vi "SphereStripSection.vi"(0 "Ducer":cluster{"radius":dbl, "h":dbl, "l":dbl} {"radius" format="%.2f"; "l" format="%.2f"; "h" format="%.2f"}, 2 "Rotate":dbl format="%.2f") -> (1 "thetas":dbl[](array[numeric]) format="%.2f", 4 "phis":dbl[](array[numeric]) format="%.2f", 6 "x matrix":dbl[][](array[numeric]) format="%.2f", 7 "y matrix":dbl[][](array[numeric]) format="%.2f", 8 "z matrix":dbl[][](array[numeric]) format="%.2f")   [LabVIEW 2022 SP3]
uses:
  <vilib>/Analysis/NI_AALPro.lvlib
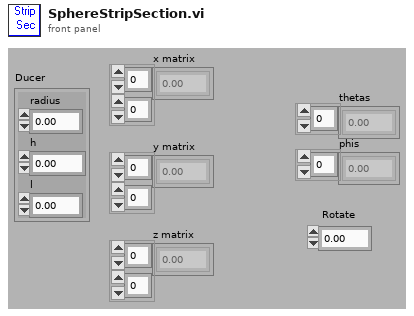
[diagram p1: front panel]
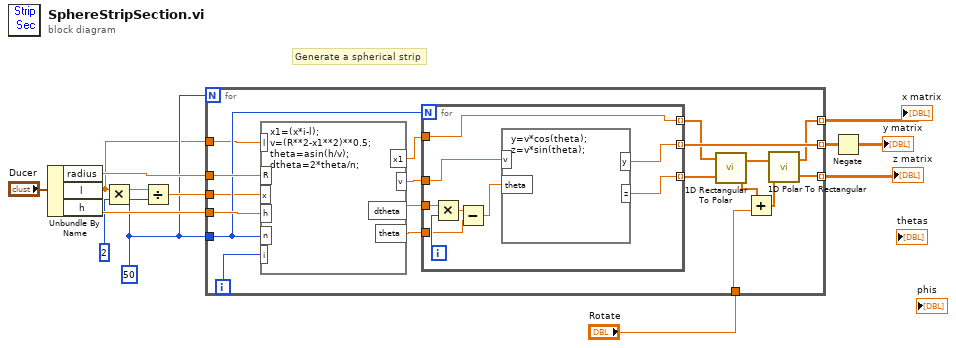
[diagram p0: block diagram]
diagram:
  w9 = 50
  # "Generate a spherical strip"
  n1 = Unbundle By Name("Ducer") -> ("radius"=w11:dbl, "l"=w3:dbl, "h"=w10:dbl)
  n2 = Multiply(x=w3, y=2) -> (x*y=w5:dbl)
  n3 = Divide(x=w5, y=w9) -> (x/y=w12:dbl)
  n4 = for {
    N: w9 -> [_]
    tunnel: [w14] -> w8 mode=indexing
    tunnel: [w16] -> w7 mode=indexing
    tunnel: [w17] -> w6 mode=indexing
    tunnel: w12 -> [w25]
    tunnel: w11 -> [w32]
    tunnel: w10 -> [w31]
    tunnel: w9 -> [w30]
    tunnel: w3 -> [w23]
    tunnel: "Rotate" -> [w18]
    i -> [w26]
    n5 = formula code="x1=(x*i-l);\nv=(R**2-x1**2)**0.5;\ntheta=asin(h/v);\ndtheta=2*theta/n;"("R"=w32, "x"=w25, "h"=w31, "n"=w30, "i"=w26, "l"=w23) -> ("v"=w27:dbl, "dtheta"=w29:dbl, "theta"=w28:dbl, "x1"=w24:dbl)
    n6 = for {
      N: w30 -> [_]
      tunnel: [w34] -> w15 mode=indexing
      tunnel: [w41] -> w16 mode=indexing
      tunnel: [w40] -> w22 mode=indexing
      tunnel: w29 -> [w38]
      tunnel: w28 -> [w36]
      tunnel: w24 -> [w34]
      tunnel: w27 -> [w33]
      i -> [w39]
      n7 = Multiply(x=w38, y=w39) -> (x*y=w37:dbl)
      n8 = Subtract(x=w37, y=w36) -> (x-y=w35:dbl)
      n9 = formula code="y=v*cos(theta);\nz=v*sin(theta);"("v"=w33, "theta"=w35) -> ("y"=w41:dbl, "z"=w40:dbl)
    }
    n10 = call <vilib>:"1D Rectangular To Polar.vi"("X"=w15, "Y"=w22) -> ("Magnitude"=w21:dbl[], "Phase"=w20:dbl[])  [unwired: 1 out]
    n11 = Add(x=w20, y=w18) -> (x+y=w19:dbl[])
    n12 = call <vilib>:"1D Polar To Rectangular.vi"("Magnitude"=w21, "Phase"=w19) -> ("X"=w14:dbl[], "Y"=w17:dbl[])  [unwired: 1 out]
  }
  "z matrix" <- w6
  "x matrix" <- w8
  n13 = Negate(x=w7) -> (-x=→"y matrix":dbl[][])
